vi "Overlay Delete Elements in Cluster Tree.vi"(11 "Tree Ref":refnum<vi>) -> (3 "Tree Ref Out":refnum<vi>)   [LabVIEW 2023]
panel:
  in  "Tree":string[](tree)
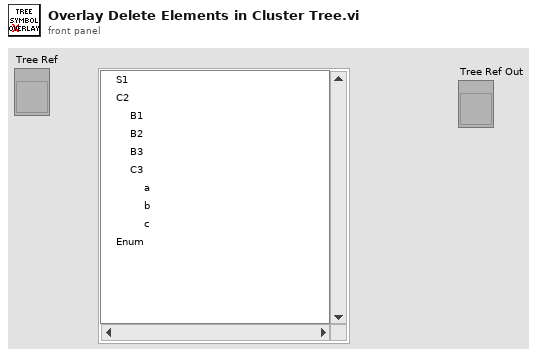
[diagram p1: front panel]
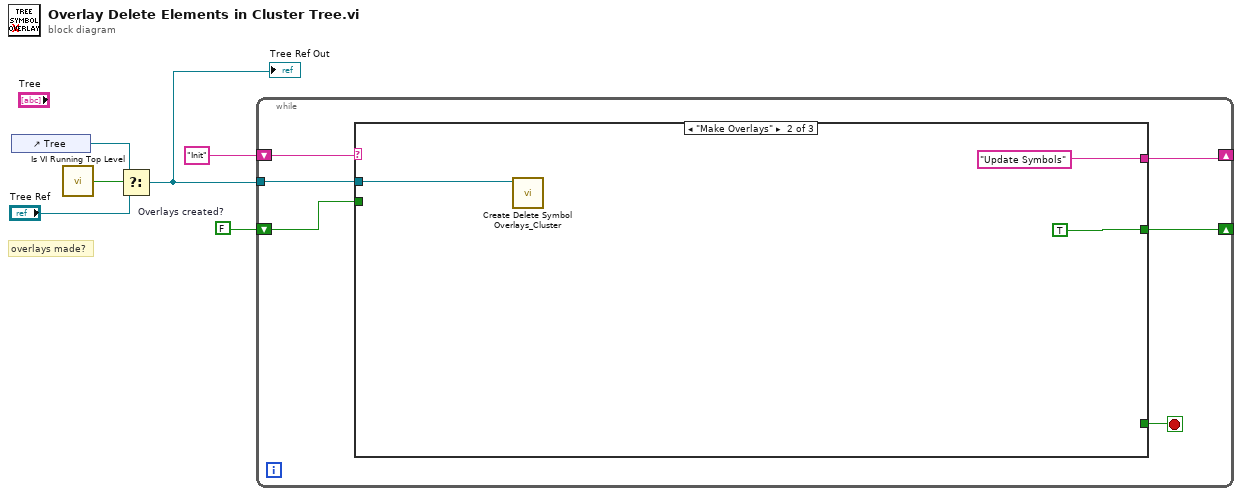
[diagram p0: block diagram]
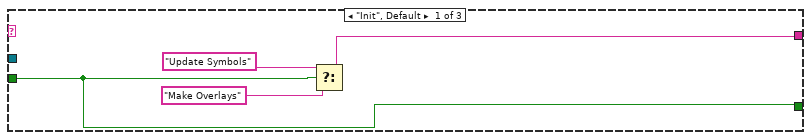
[diagram p2: hidden frame]
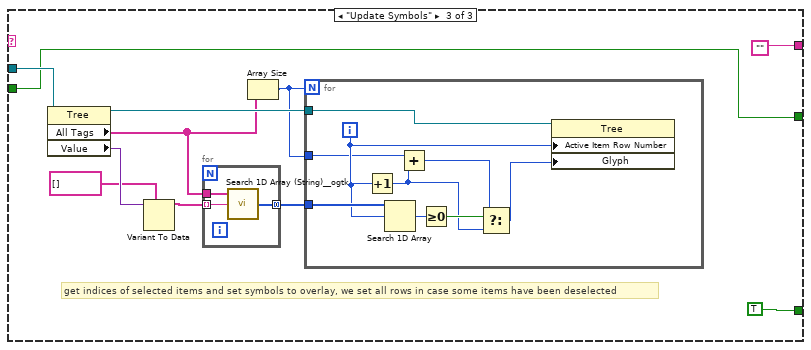
[diagram p3: hidden frame]
diagram:
  w2 = FALSE  # Overlays created?
  # "overlays made?"
  n1 = control-ref of="Tree"() -> (w5:refnum<vi>)
  n2 = call "Is VI Running Top Level.vi"() -> ("Top Level?"=w6:bool)  [unwired: 5 in]
  n3 = Select(t=w5, s=w6, f="Tree Ref") -> (s? t:f=w1:refnum<vi>)
  "Tree Ref Out" <- w1
  n4 = while {
    tunnel: w1 -> [w12]
    shift-right: [w10] -> _
    shift-left: "Init" -> [w11]
    shift-right: [w9] -> _
    shift-left: w2 -> [w8]
    stop <- w7 stop-if-true
    n5 = case shown="\"Make Overlays\"" w11 {
      tunnel: w12 -> [_ w17 w30]
      tunnel: w8 -> [w13 _ w26]
      tunnel: [w16 "Update Symbols" ""] -> w10
      tunnel: [w13 TRUE w26] -> w9
      tunnel: [_ _ TRUE] -> w7
      frame "Init", Default {
        n6 = Select(t="Update Symbols", s=w13, f="Make Overlays") -> (s? t:f=w16:string)
      }
      frame "Make Overlays" {
        n7 = call "Create Delete Symbol Overlays_Cluster.vi"("Tree Ref"=w17) -> ()  [unwired: 11 in]
      }
      frame "Update Symbols" {
        # "get indices of selected items and set symbols to overlay, we set all rows in case some items have been deselected"
        n8 = property class="Tree"(reference=w30) -> (reference out=w29:refnum<vi>, "All Tags"=w27:string[], "Value"=w23:variant)  [unwired: 1 in, 1 out]
        n9 = Variant To Data(type=string[] [], Variant=w23) -> (data=w22:string[])  [unwired: 1 in, 1 out]
        n10 = for {
          tunnel: w22 -> [w33] mode=indexing
          tunnel: [w32] -> w28 mode=concatenating
          tunnel: w27 -> [w31]
          n11 = call <userlib>:"Search 1D Array (String)__ogtk.vi"("Array"=w31, "Element Data"=w33) -> ("Indices of Elements"=w32:i32[])  [unwired: 7 in]
        }
        n12 = Array Size(array=w27) -> (size(s)=w20:i32)
        n13 = for {
          N: w20 -> [_]
          tunnel: w29 -> [w40]
          tunnel: w28 -> [w42]
          tunnel: w20 -> [w34]
          i -> [w36]
          n14 = Increment(x=w36) -> (x+1=w37:i32)
          n15 = Search 1D Array(1D array=w42, element=w36) -> (index of element=w39:i32)  [unwired: 1 in]
          n16 = Add(x=w34, y=w37) -> (x+y=w38:i32)
          n17 = Greater Or Equal To 0?(x=w39) -> (x >= 0?=w41:bool)
          n18 = Select(t=w38, s=w41, f=w37) -> (s? t:f=w35:i32)
          n19 = property class="Tree"(reference=w40, "Active Item Row Number"=w36, "Glyph"=w35) -> ()  [unwired: 1 in, 2 out]
        }
      }
    }
  }
